vi "Set Value.vi"(7 "Light Selection":T2, 8 "error in (no error)":errorcluster, 9 "Value":dbl, 10 "Update Type":T1, 11 "LightsPanel in":refnum<class "LightsPanel.lvclass">) -> (0 "error out":errorcluster, 3 "LightsPanel out":refnum<class "LightsPanel.lvclass">)   [LabVIEW 2022 SP3, in "TouchControl.lvlib" / "LightsPanel.lvclass"]
uses:
  LightsPanel.lvclass
  LightsPanel.lvclass/LightsPanel.ctl
  Update Type.ctl
  Light Selection.ctl
  TouchControl.lvlib
  Update.ctl
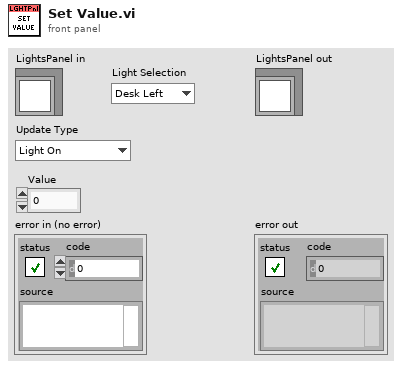
[diagram p1: front panel]
types:
  T1 = typedef "TouchControl.lvlib/LightsPanel.lvclass/Update Type.ctl" = enum16{"Light On", "Temp", "Brightness"}
  T2 = typedef "TouchControl.lvlib/Light Selection.ctl" = enum16{"Desk Left", "Desk Right", "Printer"}
  T3 = typedef "TouchControl.lvlib/LightsPanel.lvclass/Update.ctl" = cluster{"Type":T1, "Light Selection":T2, "New Value":dbl}
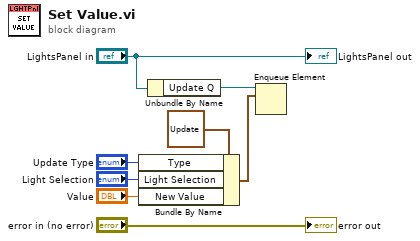
[diagram p0: block diagram]
diagram:
  n1 = Bundle By Name(cluster=T3 {"Type"=enum."Light On", "Light Selection"=enum."Desk Left", "New Value"=0.0} ("element"), "Type"="Update Type", "Light Selection"="Light Selection", "New Value"="Value") -> (w4:T3)
  n2 = Unbundle By Name("LightsPanel in") -> ("Update Q"=w6:refnum<queue>)
  n3 = Enqueue Element(queue=w6, element=w4) -> ()  [unwired: 2 in, 3 out]
  "error out" <- "error in (no error)"
  "LightsPanel out" <- "LightsPanel in"
